vi "Stop Core.vi"(10 "final error code":i32, 11 "Viewer in":refnum<class "Viewer.lvclass">) -> (3 "Viewer out":refnum<class "Viewer.lvclass">)   [LabVIEW 2015, in "Viewer.lvlib" / "Viewer.lvclass"]
doc: "(<B>Filename</B>: Actor Framework.lvlib:Actor.lvclass:Stop Core.vi)\n\nDefines what the actor does before it stops. Use the <B>final error code</B> input to determine whether the actor shut down in response to an error.\n\nBy default, this method does nothing. A descendant class may override it to define behavior, such as shutting down any processes the actor initiated in its override of the Actor Core method."
uses:
  Viewer.lvclass
  UI Window/UI Window.lvclass
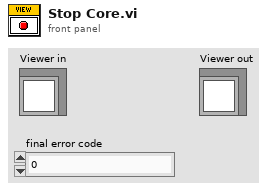
[diagram p1: front panel]
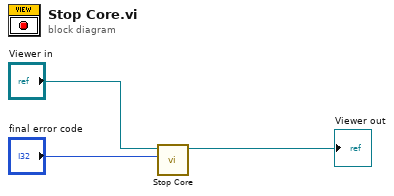
[diagram p0: block diagram]
diagram:
  n1 = call-parent "Stop Core.vi"("final error code"="final error code", "UI Window in"="Viewer in") -> ("UI Window out"=→"Viewer out":refnum<class "Viewer.lvclass">)  [unwired: 9 in]
